vi "Select Channel.vi"(8 "error in (no error)":errorcluster, 10 "Channel (1)":u32(ring)=1 items=["1"=1, "2"=2, "3"=3, "4"=4], 11 "VISA resource name":refnum<visa-resource-name>) -> (0 "error out":errorcluster, 3 "VISA resource name out":refnum<visa-resource-name>)   [LabVIEW 2015, in "Fluke 28x Series.lvlib"]
doc: "Selects from channels 1 to 4 (on the 282, the choices are channels 1 and 2). Once selected, any following changes will apply to this channel alone. \n\n<b>Note:</b> This VI only applies to multichannel instruments, i.e. 282 and 284."
uses:
  <instrlib>/Fluke 28x Series/Fluke 28x Series.lvlib
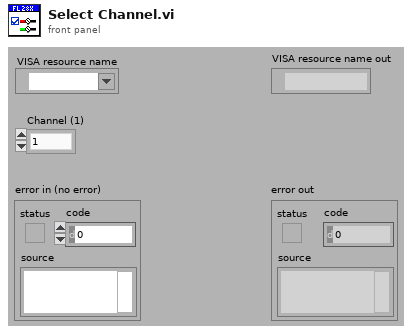
[diagram p1: front panel]
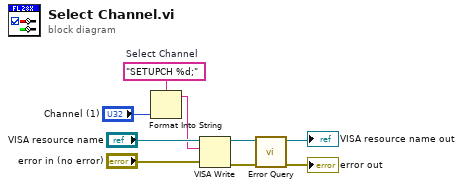
[diagram p0: block diagram]
diagram:
  w7 = "SETUPCH %d;"  # Select Channel
  n1 = Format Into String(format string=w7, "Channel (1)") -> (resulting string=w6:string)  [unwired: 2 in, 1 out]
  n2 = VISA Write(VISA resource name="VISA resource name", write buffer=w6, error in (no error)="error in (no error)") -> (VISA resource name out=w5:refnum<visa-resource-name>, error out=w4:errorcluster)  [unwired: 1 out]
  n3 = call <instrlib>:"Error Query.vi"("error in (no error)"=w4, "VISA resource name"=w5) -> ("error out"=→"error out":errorcluster, "VISA resource name out"=→"VISA resource name out":refnum<visa-resource-name>)  [unwired: 6 in, 2 out]
